vi "write-video-header-file.vi"(0 "Frames Acquired":u32, 1 "TTB Array (ms)":u32[](array[numeric]), 2 "Header2 file data":T1, 3 "time of 1st frame, \nsec":dbl format="%.2f", 5 "Sequence files handle":T3, 7 "Element 0 of TTB":u32, 9 "Pixel depth\n(0=8 bit; 1= 16 bit)":T2(ring), 11 "Error In":errorcluster, 12 "File Offsets Array":cluster{"offset":i32, "file number":u8}[](array[cluster]), 13 "Region width":i32, 14 "Region height":i32) -> (15 "Error Out":errorcluster)   [LabVIEW 2014]
uses:
  ctt's/Header2 file.ctl
  ctt's/header1 file.ctl
  File Directory/File-Locations-Global.vi
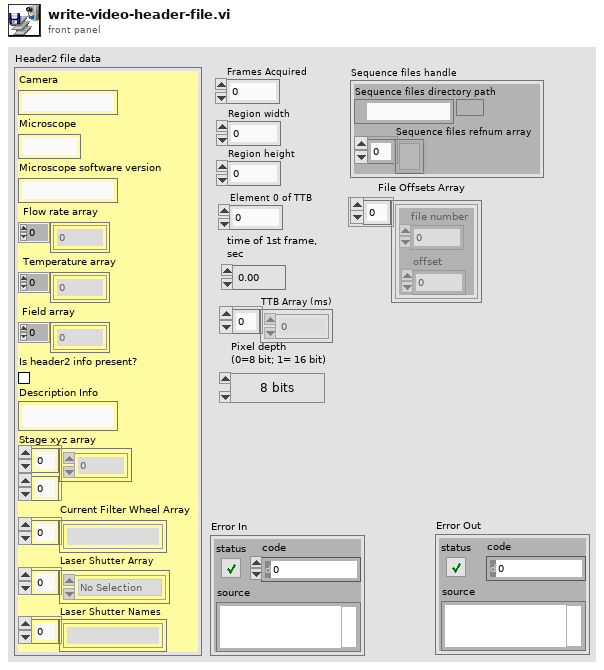
[diagram p1: front panel]
types:
  T1 = typedef "Header2 file.ctl" = cluster{"Camera":string, "Microscope":string, "Microscope software version":string, "Flow rate array":dbl[], "Temperature array":dbl[], "Field array":u16[], "Is header2 info present?":bool, "Description Info":string, "Stage xyz array":dbl[][], "Current Filter Wheel Array":string[], "Laser Shutter Array":enum32{"No Selection", "GFP", "Cy3 Long \nPass", "Cy3", "Cy5", "Off", "IR"}[], "Laser Shutter Names":string[]}
  T2 = enum16{"8 bits", "16 bits", "Float", "Complex", "RGB", "HSL"}
  T3 = cluster{"Sequence files directory path":path, "Sequence files refnum array":refnum<file>[]}
  T4 = enum16{"open", "replace", "create", "open or create", "replace or create", "replace or create with confirmation"}
  T5 = typedef "header1 file.ctl" = cluster{"Frames Acquired":u32, "Region width":i32, "Region height":i32, "Element 0 of TTB":u32, "time of 1st frame, \nsec":dbl, "TTB Array (ms)":u32[], "Offsets Array":cluster{"offset":i32, "file number":u8}[], "Pixel depth":u32}
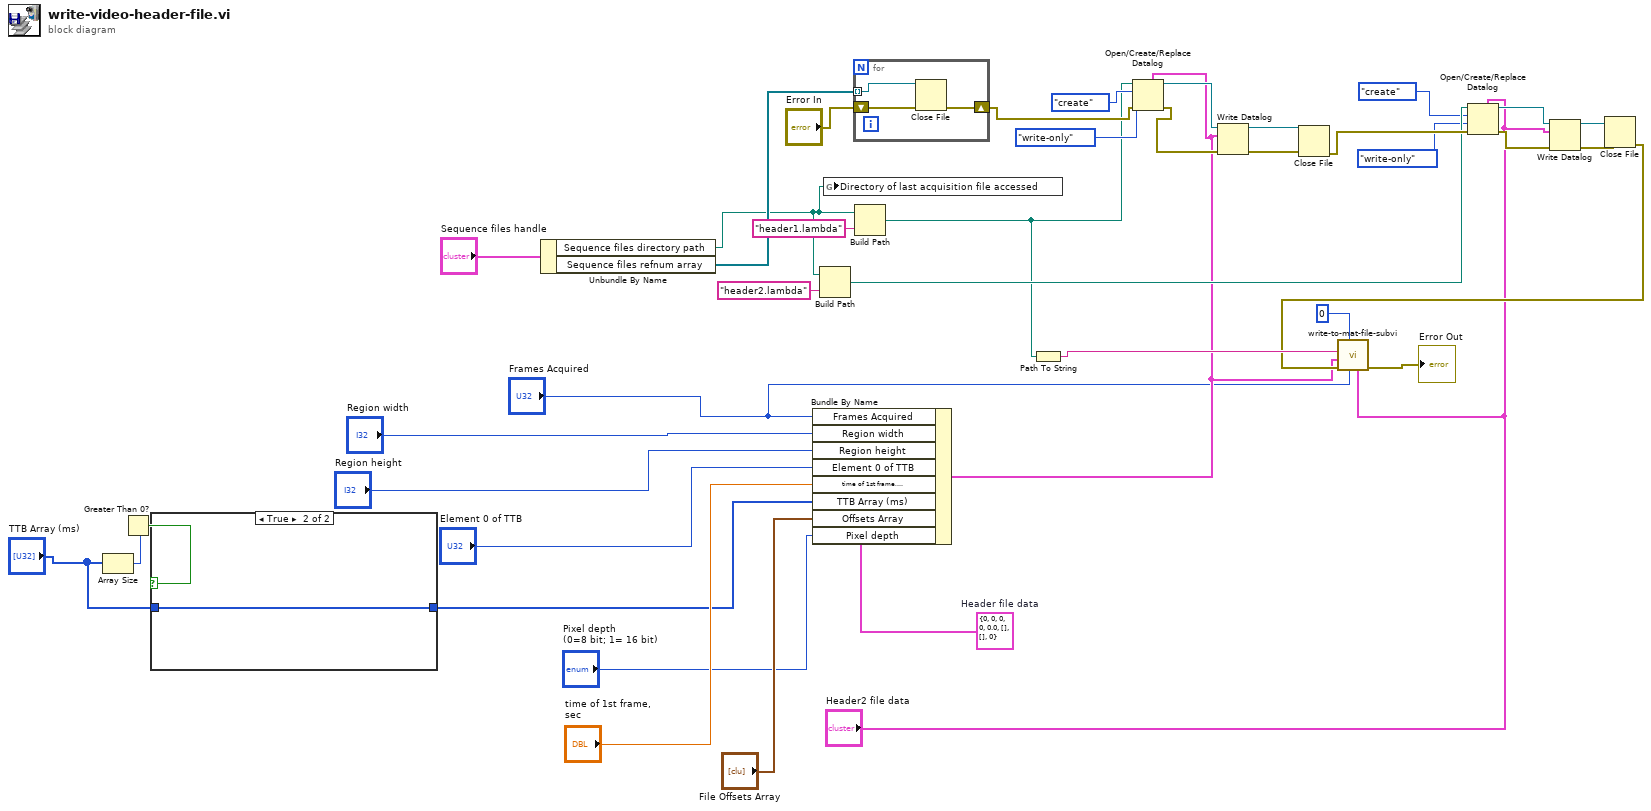
[diagram p0: block diagram]
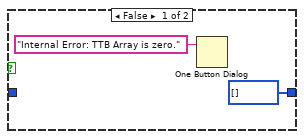
[diagram p2: hidden frame]
diagram:
  w39 = T5 {"Frames Acquired"=0, "Region width"=0, "Region height"=0, "Element 0 of TTB"=0, "time of 1st frame, \nsec"=0.0, "TTB Array (ms)"=[], "Offsets Array"=[], "Pixel depth"=0}  # Header file data
  n1 = Array Size(array="TTB Array (ms)") -> (size(s)=w33:i32)
  n2 = Greater Than 0?(x=w33) -> (x > 0?=w32:bool)
  n3 = case shown="True" w32 {
    tunnel: [u32[] [] ("TTB Array (ms)") w43] -> w30
    tunnel: "TTB Array (ms)" -> [_ w43]
    frame False {
      n4 = One Button Dialog(message="Internal Error: TTB Array is zero.") -> ()  [unwired: 1 in, 1 out]
    }
    frame True {
    }
  }
  n5 = Unbundle By Name("Sequence files handle") -> ("Sequence files directory path"=w28:path, "Sequence files refnum array"=w29:refnum<file>[])
  n6 = Bundle By Name(cluster=w39, "Frames Acquired"="Frames Acquired", "Region width"="Region width", "Region height"="Region height", "Element 0 of TTB"="Element 0 of TTB", "time of 1st frame, \nsec"="time of 1st frame, \nsec", "TTB Array (ms)"=w30, "Offsets Array"="File Offsets Array", "Pixel depth"="Pixel depth\n(0=8 bit; 1= 16 bit)") -> (w4:T5)
  n7 = Build Path(base path=w28, name or relative path="header2.lambda") -> (appended path=w17:path)
  n8 = global write "File-Locations-Global.vi" "Directory of last acquisition file accessed"(w28) -> ()
  n9 = for {
    tunnel: w29 -> [w46] mode=indexing
    shift-right: [w44] -> w24
    shift-left: "Error In" -> [w45]
    n10 = Close File(refnum=w46, error in=w45) -> (error out=w44:errorcluster)  [unwired: 1 out]
  }
  n11 = Build Path(base path=w28, name or relative path="header1.lambda") -> (appended path=w10:path)
  n12 = Path To String(path=w10) -> (string=w8:string)
  n13 = Open/Create/Replace Datalog(5:w4, 8:w24, 9:enum16{"read/write", "read-only", "write-only"}."write-only" ("access (0:read/write)"), 10:T4."create" ("operation (0:open)"), 11:w10) -> (0:w25:errorcluster, 3:w21:refnum<k1>)  [unwired: 1 in, 1 out]
  n14 = Write Datalog(4:w25, 6:w4, 7:w21) -> (0:w20:errorcluster, 3:w19:refnum<k1>)
  n15 = Close File(refnum=w19, error in=w20) -> (error out=w18:errorcluster)  [unwired: 1 out]
  n16 = Open/Create/Replace Datalog(5:"Header2 file data", 8:w18, 9:enum16{"read/write", "read-only", "write-only"}."write-only" ("access (0:read/write)"), 10:T4."create" ("operation (0:open)"), 11:w17) -> (0:w13:errorcluster, 3:w14:refnum<k1>)  [unwired: 1 in, 1 out]
  n17 = Write Datalog(4:w13, 6:"Header2 file data", 7:w14) -> (0:w12:errorcluster, 3:w11:refnum<k1>)
  n18 = Close File(refnum=w11, error in=w12) -> (error out=w7:errorcluster)  [unwired: 1 out]
  n19 = call "write-to-mat-file-subvi.vi"("Header2 file data"="Header2 file data", "Number of frames"="Frames Acquired", "first frame number"=u32 0, "Error In"=w7, "Header file data"=w4, "Movie file name"=w8) -> ("Error Out"=→"Error Out":errorcluster)  [unwired: 5 in]
